vi "Include Library.vi"(9 "Local library? (F)":bool, 10 "Library Name":string, 11 "String in":string) -> (3 "String out":string)   [LabVIEW 2014, in "C Header Generator.lvlib"]
uses:
  C Header Generator.lvlib
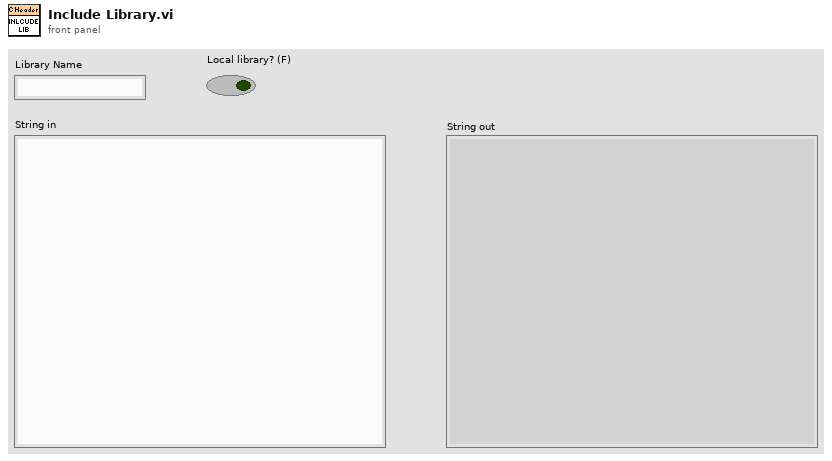
[diagram p1: front panel]
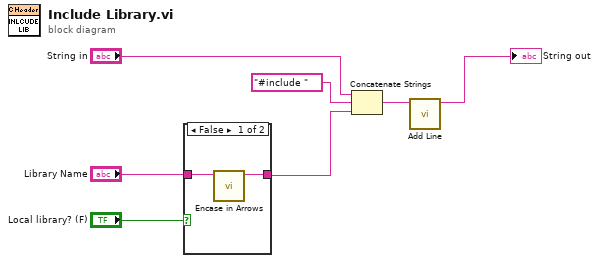
[diagram p0: block diagram]
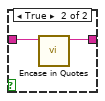
[diagram p2: hidden frame]
diagram:
  n1 = case shown="False" "Local library? (F)" {
    tunnel: "Library Name" -> [w9 w11]
    tunnel: [w8 w10] -> w1
    frame False {
      n2 = call "Encase in Arrows.vi"("String in"=w9) -> ("String out"=w8:string)  [unwired: 10 in]
    }
    frame True {
      n3 = call "Encase in Quotes.vi"("String in"=w11) -> ("String out"=w10:string)  [unwired: 10 in]
    }
  }
  n4 = Concatenate Strings("String in", "#include ", w1) -> (w5:string)
  n5 = call "Add Line.vi"("String in"=w5) -> ("String out"=→"String out":string)  [unwired: 10 in]
